vi "CHECKSN_SFC.vi"(8 "error in":errorcluster, 9 "SN":string, 10 "menu reference":refnum<k9>, 11 "OPID":string) -> (0 "error out":errorcluster, 1 "SNCheck":bool)   [LabVIEW 2013]
uses:
  Control/Buffer.vi
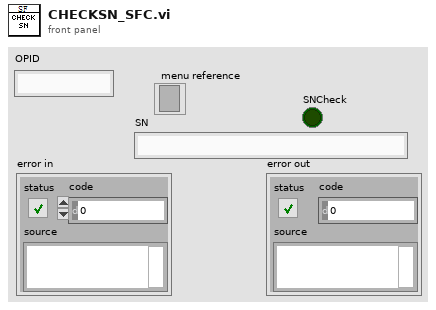
[diagram p1: front panel]
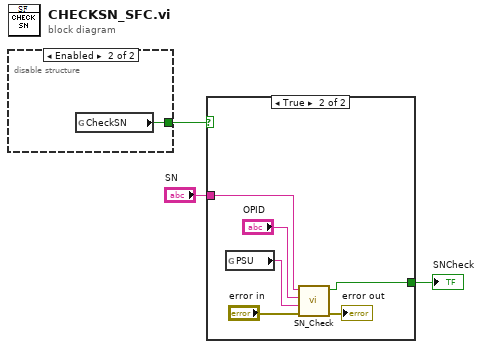
[diagram p0: block diagram]
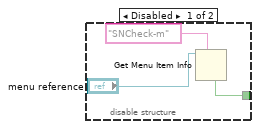
[diagram p2: hidden frame]
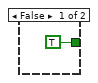
[diagram p3: hidden frame]
diagram:
  n1 = disable-structure shown="Enabled" {
    disable-tunnel: [w5 w7] -> w1
    frame Disabled {
      n2 = Get Menu Item Info(7:"SNCheck-m" ("item tag"), 11:"menu reference") -> (4:w5:bool)  [unwired: 1 in, 6 out]
    }
    frame Enabled {
      n3 = global read "Buffer.vi" "CheckSN"() -> (w7:bool)
    }
  }
  n4 = case shown="True" w1 {
    tunnel: [TRUE w12] -> w3
    tunnel: "SN" -> [_ w14]
    frame False {
    }
    frame True {
      n5 = global read "Buffer.vi" "PSU"() -> (w9:string)
      n6 = call "SN_Check.vi"("error in"="error in", "PSU"=w9, "OPID"="OPID", "SN"=w14) -> ("error out"=→"error out":errorcluster, "pass?"=w12:bool)  [unwired: 6 in]
    }
  }
  "SNCheck" <- w3
